vi "Launcher.vi"(8 "error in (no error)":errorcluster, 9 "VideoQueue":refnum<queue>, 10 "ResponseNotifier":refnum<notifier>, 11 "CamParameters":T1) -> (0 "error out":errorcluster)   [LabVIEW 2020, in "CameraTestingProxy.lvlib" / "CameraTestingENI.lvclass"]
uses:
  CameraTestingENI.lvclass
  Camera/ICamera/ICamera/ICamera.lvclass
  ICameraTestingProxy/ICameraTestingProxy/TypeDef/VideoFrameData.ctl
  C:/Program Files (x86)/National Instruments/LabVIEW 2020/vi.lib/ActorFramework/Actor/Actor.lvclass
  CameraTestingENI.lvclass/CameraTestingENI.ctl
  <vilib>/ActorFramework/Message Enqueuer/Message Enqueuer.lvclass/Message Enqueuer.ctl
  <vilib>/ActorFramework/Message Enqueuer/Enqueue.vi
  CameraTestingENI Messages/Init Msg/Init Msg.lvclass
  C:/Program Files (x86)/National Instruments/LabVIEW 2020/vi.lib/ActorFramework/Message/Message.lvclass
  CameraTestingENI Messages/GetEvents Msg/GetEvents Msg.lvclass
  <vilib>/ActorFramework/Message Priority Queue/Priority Enqueue.vi
  <vilib>/ActorFramework/Actor/Actor.lvclass
  ICameraTestingProxy/ICameraTestingProxy/ICameraTestingProxy.lvclass
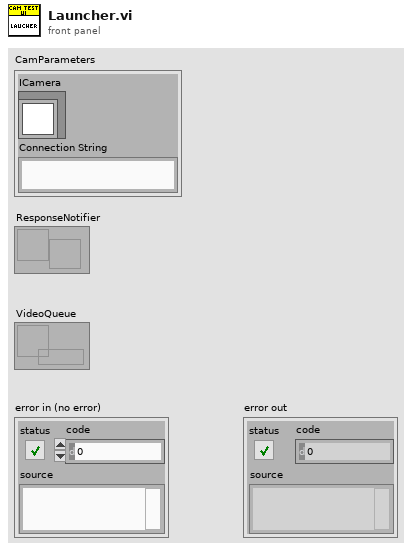
[diagram p1: front panel]
types:
  T1 = cluster{"ICamera":refnum<class "ICamera.lvclass">, "Connection String":string}
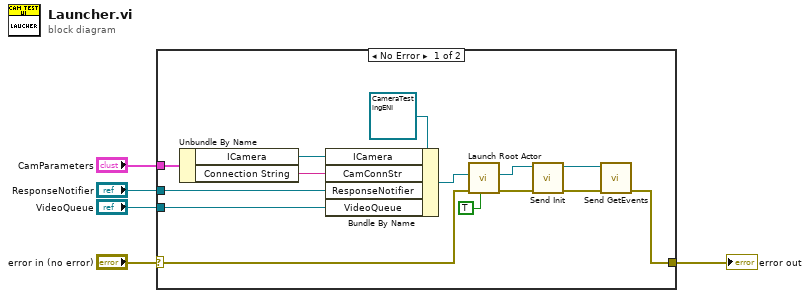
[diagram p0: block diagram]
diagram:
  n1 = case shown="No Error" "error in (no error)" {
    selector: "error in (no error)" -> [w9 w20]
    tunnel: "CamParameters" -> [w18 _]
    tunnel: "ResponseNotifier" -> [w15 _]
    tunnel: [w8 w20] -> w2
    tunnel: "VideoQueue" -> [w7 _]
    frame No Error {
      n2 = Unbundle By Name(w18) -> ("ICamera"=w17:refnum<class "ICamera.lvclass">, "Connection String"=w16:string)
      n3 = Bundle By Name(cluster=refnum<class "CameraTestingENI.lvclass"> refnum ("CameraTestingProxy.lvlib:CameraTestingTRXI.lvclass"), "ICamera"=w17, "CamConnStr"=w16, "ResponseNotifier"=w15, "VideoQueue"=w7) -> (w14:refnum<class "CameraTestingENI.lvclass">)
      n4 = call <vilib>:"Launch Root Actor.vi"("Open Actor Core front panel? (F)"=TRUE, "error in (no error)"=w9, "Actor"=w14) -> ("error out"=w12:errorcluster, "Actor's Enqueuer"=w13:refnum<class "Message Enqueuer.lvclass">)  [unwired: 7 in]
      n5 = call "Send Init.vi"("error in (no error)"=w12, "Message Enqueuer"=w13) -> ("error out"=w11:errorcluster, "Message Enqueuer out"=w10:refnum<class "Message Enqueuer.lvclass">)  [unwired: 8 in]
      n6 = call "Send GetEvents.vi"("error in (no error)"=w11, "Message Enqueuer"=w10) -> ("error out"=w8:errorcluster)  [unwired: 8 in, 1 out]
    }
    frame Error {
    }
  }
  "error out" <- w2
